vi "CV.vi"() -> ()   [LabVIEW 2023]
uses:
  Sub_Vi/TypeDefsControls/Voltage.ctl
  Sub_Vi/TypeDefsControls/Iterator.ctl
  Sub_Vi/TypeDefs/WayPointCluster.ctl
  Sub_Vi/TypeDefs/ChangeOnFly.ctl
  Sub_Vi/TypeDefs/Settings.ctl
  Sub_Vi/TypeDefs/Display.ctl
  Sub_Vi/TypeDefsControls/Voltage Scan Rate.ctl
  Sub_Vi/TypeDefsControls/Time.ctl
  Settings.vi
panel:
  out "V vs C2":cluster{"Y":dbl[], "Y":dbl[]}[](graph)
  in  "Output Channel":u16(ring) items=["Voltage 1 (AO3)", "Voltage 2 (AO4)"]
  in  "Quiet Time (s)":T1 min=0.0
  in  "Scan Rate (V/s)":T2=0.2 min=0.0 max=1000.0
  in  "Second Voltage (V)":T3=1.0 min=-10.0 max=10.0
  in  "First Voltage (V)":T3=-1.0 min=-10.0 max=10.0
  in  "Start scan Button":bool
  in  "Jump at Start":bool
  in  "Display Cluster":T4
  in  "SettingsCluster":T5={"Sample Rate (us)"=1, "Samples Per Data Point (int, power of 2)"=1000, "DistanceToBulk (um)"=-1.0, "HoldTimeScaler"=1, "SaveData"=TRUE, "DistanceToBulk (um) 2"=-1.0, "DistanceToBulk (um) 3"=-1.0}
  in  "ChangeonFly":T6
  in  "WayPointCluster":T7
  in  "Number of Cycles":T8=1.0 min=1.0
  in  "Start Voltage (V)":T3 min=-10.0 max=10.0
  in  "stop":bool
  # "Settings"
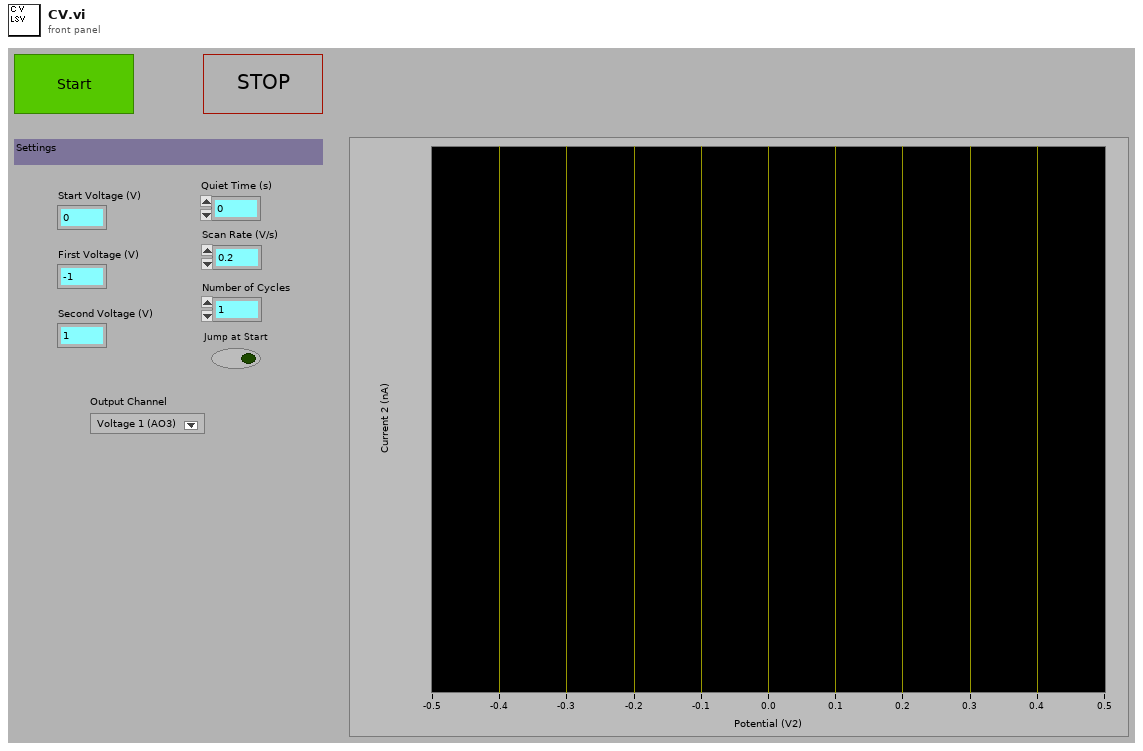
[diagram p1: front panel]
types:
  T1 = typedef "Time.ctl" = dbl
  T2 = typedef "Voltage Scan Rate.ctl" = dbl
  T3 = typedef "Voltage.ctl" = dbl
  T4 = typedef "Display.ctl" = cluster{"X":refnum<vi>, "Y":refnum<vi>, "Z":refnum<vi>, "Amp":refnum<vi>, "Phase":refnum<vi>, "t vs Z":refnum<vi>, "t vs C1":refnum<vi>, "t vs C2":refnum<vi>, "t vs C3":refnum<vi>, "t vs Amp":refnum<vi>, "t vs Phase":refnum<vi>, "t vs X":refnum<vi>, "t vs Y":refnum<vi>, "Z vs C1":refnum<vi>, "Z vs C2":refnum<vi>, "Z vs C3":refnum<vi>, "V vs C1":refnum<vi>, "V vs C2":refnum<vi>, "V vs C3":refnum<vi>, "X/Y/Z F":refnum<vi>, "X/Y/Z R":refnum<vi>, "X/Y/C1 F":refnum<vi>, "X/Y/C1 R":refnum<vi>, "X/Y/C2 F":refnum<vi>, "X/Y/C2 R":refnum<vi>, "X/Y/C3 F":refnum<vi>, "X/Y/C3 R":refnum<vi>, "NumberOfLines":u16, "um Per Pixel":dbl, "um Per Line":dbl, "X Center":dbl, "Hop X/Y/Z":refnum<vi>, "Hop X/Y/C1":refnum<vi>, "Hop X/Y/C2":refnum<vi>, "Hop X/Y/C3":refnum<vi>, "X Width":dbl, "Y Width":dbl, "Hopping Distance":dbl, "V2 vs C1":refnum<vi>, "V vs Phase":refnum<vi>, "Y Center":dbl, "Number of Pixels":dbl, "V2 vs C2":refnum<vi>, "V2 vs C3":refnum<vi>, "V vs y":refnum<vi>, "V2 vs y":refnum<vi>, "Z vs Amp":refnum<vi>, "Z vs Phase":refnum<vi>}
  T5 = typedef "Settings.ctl" = cluster{"Sample Rate (us)":u32, "Samples Per Data Point (int, power of 2)":i16, "DistanceToBulk (um)":dbl, "HoldTimeScaler":u64, "SaveData":bool, "DistanceToBulk (um) 2":dbl, "DistanceToBulk (um) 3":dbl}
  T6 = typedef "ChangeOnFly.ctl" = cluster{"Stop (boolean)":refnum<vi>, "Pause (boolean)":refnum<vi>, "EndCurrentLine (boolean)":refnum<vi>, "max movement per update step (Interger, nm)":refnum<vi>, "P (float, arb)":refnum<vi>, "Feedback set point (double, Amps)":refnum<vi>, "Voltage (double, V)":refnum<vi>, "Feedback set point 2 (double, Amps)":refnum<vi>, "Stop on Greater Than 2? (boolean)":refnum<vi>, "Stop on Greater Than? (boolean)":refnum<vi>, "Voltage 2 (double, V)":refnum<vi>, "Feedback Type (enum)":refnum<vi>, "Feedback Type 2 (enum)":refnum<vi>}
  T7 = typedef "WayPointCluster.ctl" = cluster{"X (um)":dbl[], "Y (um)":dbl[], "Z (um)":dbl[], "V (V)":dbl[], "X Velocity (um s-1)":dbl[], "Y Velocity (um s-1)":dbl[], "Z Velocity (um s-1)":dbl[], "V Velocity (V s-1)":dbl[], "FeedBack Type (enum)":u16[], "Move X (boolean)":bool[], "Move Y (boolean)":bool[], "Move Z (boolean)":bool[], "Move V (boolean)":bool[], "Jump V (boolean)":bool[], "Hold (boolean)":bool[], "Hold Time":u32[], "V2 (V)":dbl[], "Move V2":bool[], "V2 Velocity (V s-1)":dbl[], "Jump V2 (boolean)":bool[], "Update z Position delta (ms)":i16[], "Hold Feedback1":bool[], "Move Z PicoMotor":bool[], " Z PicoMotor Direction":bool[], "DIO0":bool[]}
  T8 = typedef "Iterator.ctl" = dbl
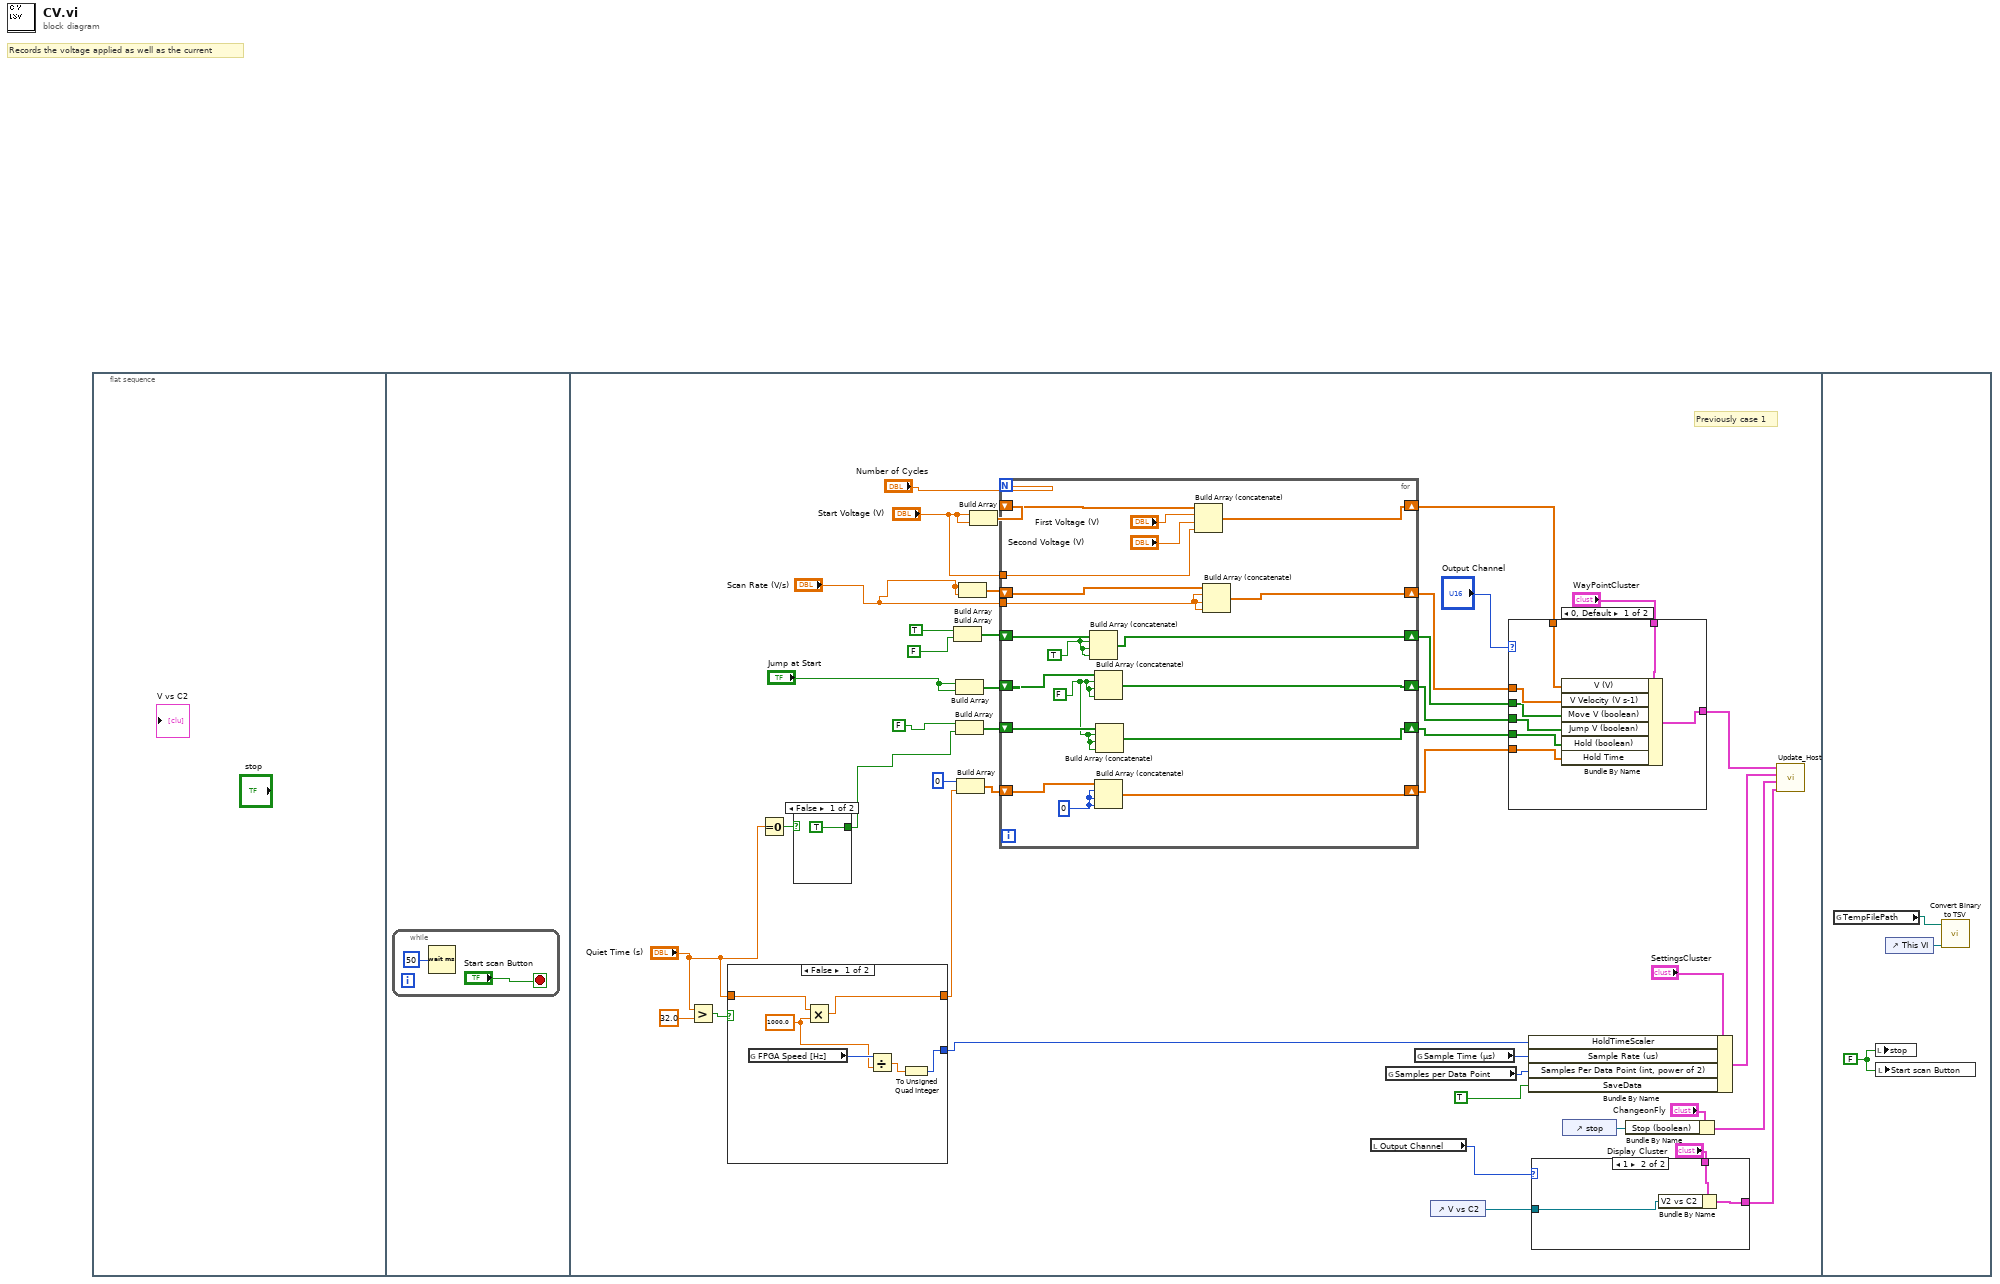
[diagram p0: block diagram]
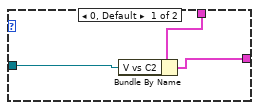
[diagram p2: hidden frame]
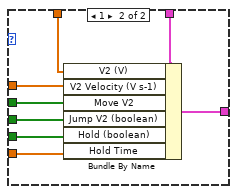
[diagram p3: hidden frame]
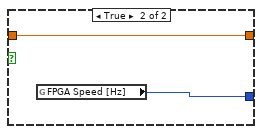
[diagram p4: hidden frame]
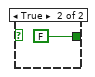
[diagram p5: hidden frame]
diagram:
  # "Records the voltage applied as well as the current"
  n1 = flat-sequence {
    frame #0 {
    }
    frame #1 {
      n2 = while {
        stop <- "Start scan Button" stop-if-true
        n3 = Wait (ms)(milliseconds to wait=u32 50) -> ()  [unwired: 1 out]
      }
    }
    frame #2 {
      # "Previously case 1"
      n4 = Greater?(x="Quiet Time (s)", y=T1 32.0) -> (0:w12:bool)
      n5 = case shown="False" w12 {
        tunnel: "Quiet Time (s)" -> [w72 w74]
        tunnel: [w71 w74] -> w10
        tunnel: [w67 w73] -> w9
        frame False {
          w69 = 1000.0 ("y")
          n6 = global read "Settings.vi" "FPGA Speed [Hz]"() -> (w70:i64)
          n7 = Multiply(x=w72, y=w69) -> (x*y=w71:T1)
          n8 = Divide(x=w70, y=w69) -> (x/y=w68:dbl)
          n9 = To Unsigned Quad Integer(1:w68) -> (0:w67:u64)
        }
        frame True {
          n10 = global read "Settings.vi" "FPGA Speed [Hz]"() -> (w73:i64)
        }
      }
      n11 = Equal To 0?(x="Quiet Time (s)") -> (x = 0?=w20:bool)
      n12 = case shown="False" w20 {
        tunnel: [TRUE ("Set Z") FALSE ("Set Z")] -> w14
        frame False {
        }
        frame True {
        }
      }
      n13 = Build Array(TRUE ("Start scan Button"), FALSE ("Start scan Button")) -> (w28:bool[])
      n14 = Build Array("Jump at Start", "Jump at Start") -> (w24:bool[])
      n15 = Build Array(FALSE ("Start scan Button"), w14) -> (w22:bool[])
      n16 = Build Array(0, w10) -> (w16:T1[])
      n17 = Build Array("Scan Rate (V/s)", "Scan Rate (V/s)") -> (w31:T2[])
      n18 = Build Array("Start Voltage (V)", "Start Voltage (V)") -> (w32:T3[])
      n19 = for {
        N: "Number of Cycles" -> [_]
        shift-right: [w94] -> w27
        shift-left: w32 -> [w95]
        shift-right: [w93] -> w26
        shift-left: w31 -> [w92]
        shift-right: [w91] -> w21
        shift-left: w24 -> [w82]
        shift-right: [w89] -> w19
        shift-left: w22 -> [w90]
        tunnel: "Start Voltage (V)" -> [w86]
        shift-right: [w84] -> w25
        shift-left: w28 -> [w85]
        shift-right: [w78] -> w15
        shift-left: w16 -> [w80]
        tunnel: "Scan Rate (V/s)" -> [w77]
        w79 = 0
        w81 = FALSE ("Start scan Button")
        w83 = TRUE ("Start scan Button")
        n20 = Build Array (concatenate)(w85, w83, w83, w83) -> (w84:bool[])
        n21 = Build Array (concatenate)(w82, w81, w81, w81) -> (w91:bool[])
        n22 = Build Array (concatenate)(w80, w79, w79, w79) -> (w78:T1[])
        n23 = Build Array (concatenate)(w90, w81, w81, w81) -> (w89:bool[])
        n24 = Build Array (concatenate)(w95, "First Voltage (V)", "Second Voltage (V)", w86) -> (w94:T3[])
        n25 = Build Array (concatenate)(w92, w77, w77, w77) -> (w93:T2[])
      }
      n26 = local read "Output Channel"() -> (w4:u16)
      n27 = global read "Settings.vi" "Samples per Data Point"() -> (w34:u16)
      n28 = global read "Settings.vi" "Sample Time (µs)"() -> (w39:u32)
      n29 = control-ref of="V vs C2"() -> (w3:refnum<vi>)
      n30 = case shown="0, Default" "Output Channel" {
        tunnel: "WayPointCluster" -> [w51 w66]
        tunnel: [w52 w65] -> w38
        tunnel: w27 -> [w58 w64]
        tunnel: w26 -> [w57 w63]
        tunnel: w25 -> [w56 w62]
        tunnel: w21 -> [w55 w61]
        tunnel: w19 -> [w54 w60]
        tunnel: w15 -> [w53 w59]
        frame 0, Default {
          n31 = Bundle By Name(cluster=w51, "V (V)"=w58, "V Velocity (V s-1)"=w57, "Move V (boolean)"=w56, "Jump V (boolean)"=w55, "Hold (boolean)"=w54, "Hold Time"=w53) -> (w52:T7)
        }
        frame 1 {
          n32 = Bundle By Name(cluster=w66, "V2 (V)"=w64, "V2 Velocity (V s-1)"=w63, "Move V2"=w62, "Jump V2 (boolean)"=w61, "Hold (boolean)"=w60, "Hold Time"=w59) -> (w65:T7)
        }
      }
      n33 = Bundle By Name(cluster="SettingsCluster", "HoldTimeScaler"=w9, "Sample Rate (us)"=w39, "Samples Per Data Point (int, power of 2)"=w34, "SaveData"=TRUE) -> (w36:T5)
      n34 = case shown="1" w4 {
        tunnel: "Display Cluster" -> [w47 w50]
        tunnel: [w46 w49] -> w37
        tunnel: w3 -> [w45 w48]
        frame 0, Default {
          n35 = Bundle By Name(cluster=w47, "V vs C2"=w45) -> (w46:T4)
        }
        frame 1 {
          n36 = Bundle By Name(cluster=w50, "V2 vs C2"=w48) -> (w49:T4)
        }
      }
      n37 = control-ref of="stop"() -> (w44:refnum<vi>)
      n38 = Bundle By Name(cluster="ChangeonFly", "Stop (boolean)"=w44) -> (w35:T6)
      n39 = call "Update_Host.vi"("Display Cluster"=w37, "ChangeonFly"=w35, "SettingsCluster"=w36, "WayPointCluster"=w38) -> ()  [unwired: 6 in]
    }
    frame #3 {
      w98 = FALSE ("Start scan Button")
      n40 = global read "Settings.vi" "TempFilePath"() -> (w96:path)
      n41 = local write "stop"(w98) -> ()
      n42 = local write "Start scan Button"(w98) -> ()
      n43 = control-ref of="This VI"() -> (w97:refnum<vi>)
      n44 = call "Convert Binary to TSV.vi"("This VI"=w97, "TDMS DataFile Name"=w96) -> ()  [unwired: 10 in]
    }
  }
